vi "Initialize Data Notifiers.vi"(8 "error in (no error)":errorcluster) -> (0 "error out":errorcluster, 3 "Notifiers Created":string[](array[string]))   [LabVIEW 2020]
doc: "This VI initilizes the data notifiers that will be used by the telemetry handler to load the most recent data onto their respective registers."
uses:
  Type Definitions/Payload Class.ctl
  Type Definitions/Enum - System State.ctl
  Type Definitions/Enum - Parameters.ctl
  Type Definitions/Enum - Metadata.ctl
  Type Definitions/Enumerated Constants/Software Monitor.ctl
  Type Definitions/Enum - Data.ctl
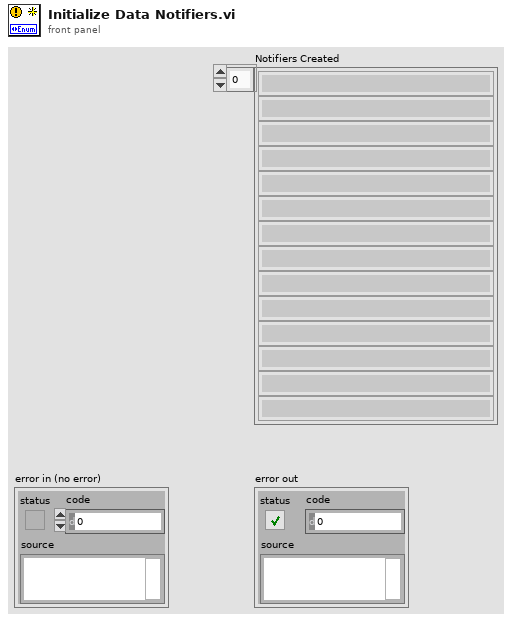
[diagram p1: front panel]
types:
  T1 = typedef "Payload Class.ctl" = enum16{"System State", "Parameters", "Metadata", "Software Monitor", "Data", "Commands"}
  T2 = typedef "Enum - System State.ctl" = enum16{"System Time", "Telemetry TCP State", "Writeable Drive State", "Command TCP State", "Network Adapter State", "Discovery Engine State", "Disk State"}
  T3 = typedef "Enum - Parameters.ctl" = enum16{"Device Parameters"}
  T4 = typedef "Enum - Metadata.ctl" = enum16{"Computer Metadata", "Computer Resources", "RT Image Metadata", "Startup Settings", "Telemetry Recorder Status"}
  T5 = typedef "Software Monitor.ctl" = enum16{"Internet Connection Monitor", "CPU Monitor", "Archive Monitor", "Memory Monitor", "Queue Monitor", "RTOS Update", "RTOS Monitor"}
  T6 = typedef "Enum - Data.ctl" = enum16{"Analog Input Data", "Notification Data", "Analog Output Data", "Digital Output Data", "Command Ack", "Digital Input Data", "GPS Solution Data"}
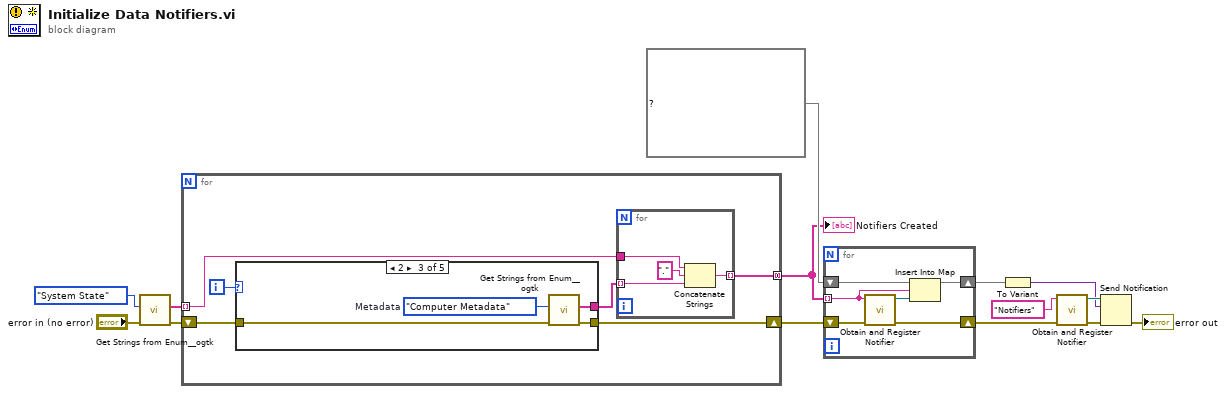
[diagram p0: block diagram]
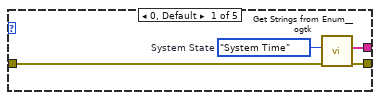
[diagram p2: hidden frame]
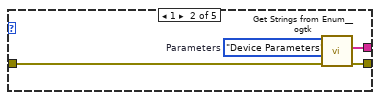
[diagram p3: hidden frame]
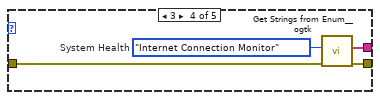
[diagram p4: hidden frame]
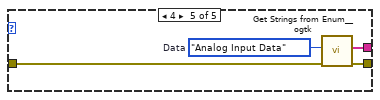
[diagram p5: hidden frame]
diagram:
  n1 = call <userlib>:"Get Strings from Enum__ogtk.vi"("error in (no error)"="error in (no error)", "Enum"=Payload_Class."System State" ("Payload Class")) -> ("error out"=w3:errorcluster, "Enum Strings"=w12:string[])  [unwired: 6 in, 2 out]
  n2 = for {
    tunnel: w12 -> [w19] mode=indexing
    tunnel: [w17] -> w5 mode=concatenating
    shift-right: [w15] -> w2
    shift-left: w3 -> [w16]
    i -> [w20]
    n3 = case shown="2" w20 {
      tunnel: [w27 w32 w36 w40 w44] -> w18
      tunnel: w16 -> [w25 w30 w34 w38 w42]
      tunnel: [w26 w29 w33 w37 w41] -> w15
      frame 0, Default {
        w28 = Enum_-_System_State."System Time"  # System State
        n4 = call <userlib>:"Get Strings from Enum__ogtk.vi"("error in (no error)"=w25, "Enum"=w28) -> ("error out"=w26:errorcluster, "Enum Strings"=w27:string[])  [unwired: 6 in, 2 out]
      }
      frame 1 {
        w31 = Enum_-_Parameters."Device Parameters"  # Parameters
        n5 = call <userlib>:"Get Strings from Enum__ogtk.vi"("error in (no error)"=w30, "Enum"=w31) -> ("error out"=w29:errorcluster, "Enum Strings"=w32:string[])  [unwired: 6 in, 2 out]
      }
      frame 2 {
        w35 = Enum_-_Metadata."Computer Metadata"  # Metadata
        n6 = call <userlib>:"Get Strings from Enum__ogtk.vi"("error in (no error)"=w34, "Enum"=w35) -> ("error out"=w33:errorcluster, "Enum Strings"=w36:string[])  [unwired: 6 in, 2 out]
      }
      frame 3 {
        w39 = Software_Monitor."Internet Connection Monitor"  # System Health
        n7 = call <userlib>:"Get Strings from Enum__ogtk.vi"("error in (no error)"=w38, "Enum"=w39) -> ("error out"=w37:errorcluster, "Enum Strings"=w40:string[])  [unwired: 6 in, 2 out]
      }
      frame 4 {
        w43 = Enum_-_Data."Analog Input Data"  # Data
        n8 = call <userlib>:"Get Strings from Enum__ogtk.vi"("error in (no error)"=w42, "Enum"=w43) -> ("error out"=w41:errorcluster, "Enum Strings"=w44:string[])  [unwired: 6 in, 2 out]
      }
    }
    n9 = for {
      tunnel: w19 -> [w24]
      tunnel: w18 -> [w22] mode=indexing
      tunnel: [w21] -> w17 mode=indexing
      n10 = Concatenate Strings(w24, "." ("string"), w22) -> (w21:string)
    }
  }
  "Notifiers Created" <- w5
  n11 = for {
    tunnel: w5 -> [w49] mode=indexing
    shift-right: [w47] -> w11
    shift-left: map{string, refnum<notifier>} {} ("map") -> [w50]
    shift-right: [w45] -> w1
    shift-left: w2 -> [w46]
    n12 = call "Obtain and Register Notifier.vi"("error in (no error)"=w46, "name (unnamed)"=w49) -> ("error out"=w45:errorcluster, "notifier out"=w48:refnum<notifier>)  [unwired: 7 in, 1 out]
    n13 = Insert Into Map(map in=w50, key=w49, value=w48) -> (map out=w47:map{string, refnum<notifier>})  [unwired: 2 out]
  }
  n14 = To Variant(anything=w11) -> (Variant=w7:variant)
  n15 = call "Obtain and Register Notifier.vi"("error in (no error)"=w1, "name (unnamed)"="Notifiers") -> ("error out"=w6:errorcluster, "notifier out"=w8:refnum<notifier>)  [unwired: 7 in, 1 out]
  n16 = Send Notification(notification=w7, notifier=w8, error in (no error)=w6) -> (error out=→"error out":errorcluster)  [unwired: 1 out]
